vi "Process Mouse Up.vi"(0 "Listbox":refnum<vi>, 1 "Ring":refnum<vi>, 5 "Rows":T1[](array[typedef]), 7 "Items":i32[](array[numeric]), 9 "Coords":T3, 11 "error in (no error)":errorcluster) -> (8 "row":i32, 15 "error out":errorcluster)   [LabVIEW 2015, in "KPropertyTable.xctl"]
uses:
  KPropertyTable.xctl
  <vilib>/Utility/miscctls.llb/LVPoint32TypeDef.ctl
  RowData.ctl
  DataType.ctl
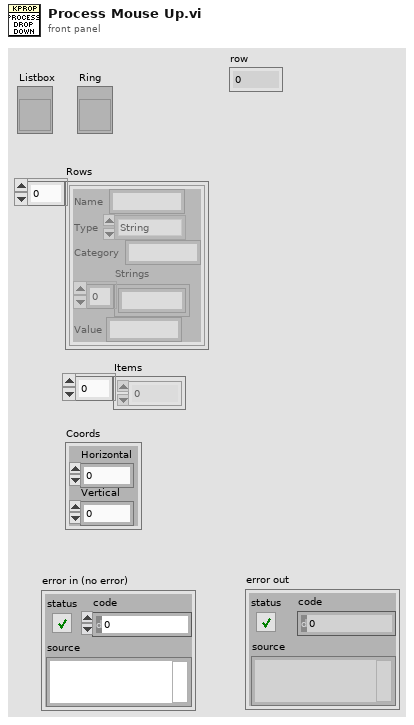
[diagram p1: front panel]
types:
  T1 = typedef "KPropertyTable.xctl/RowData.ctl" = cluster{"Name":string, "Type":T2, "Category":string, "Strings":string[], "Value":string}
  T2 = typedef "KPropertyTable.xctl/DataType.ctl" = enum16{"String", "Enum", "Int", "Double", "Boolean", "Ring", "Formula"}
  T3 = typedef "LVPoint32TypeDef.ctl" = cluster{"Horizontal":i32, "Vertical":i32}
  T4 = typedef "LVRowAndColumnTypeDef.ctl" = cluster{"Row":i32, "Column":i32}
  T5 = typedef "LVPositionTypeDef.ctl" = cluster{"Left":i32, "Top":i32}
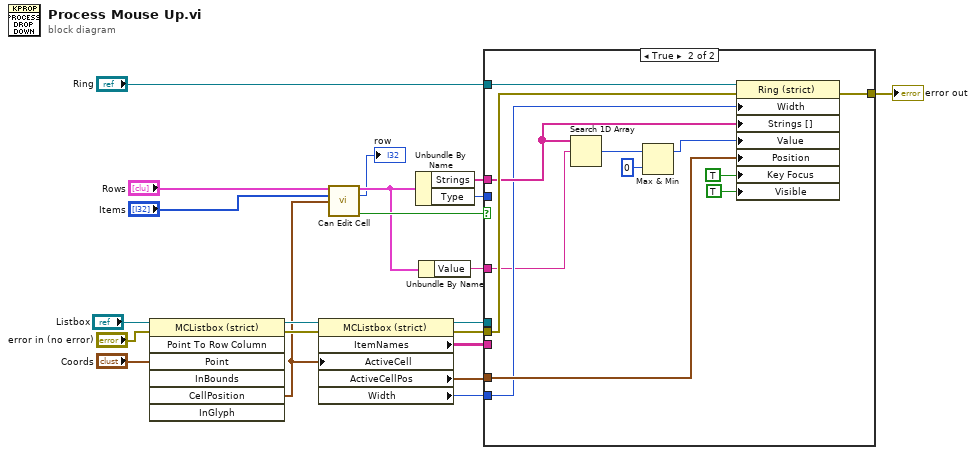
[diagram p0: block diagram]
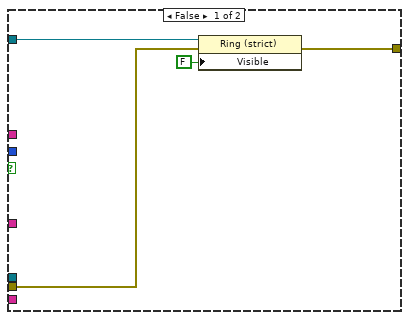
[diagram p2: hidden frame]
diagram:
  n1 = invoke on="Invoke Node" class="MCListbox (strict)" method="Point To Row Column"(reference="Listbox", error in="error in (no error)", "Point"="Coords") -> (reference out=w18:refnum<vi>, error out=w17:errorcluster, "CellPosition"=w7:T4)  [unwired: 4 in, 4 out]
  n2 = property class="MCListbox (strict)"(reference=w18, error in=w17, "ActiveCell"=w7) -> (reference out=w8:refnum<vi>, error out=w12:errorcluster, "ItemNames"=w13:string[][], "ActiveCellPos"=w15:T5, "Width"=w4:u32)
  n3 = call "Can Edit Cell.vi"("Rows"="Rows", "Items"="Items", "Cell"=w7) -> ("item"=w3:T1, "row"=→"row":i32, "enum?"=w5:bool)  [unwired: 9 in, 1 out]
  n4 = Unbundle By Name(w3) -> ("Strings"=w14:string[], "Type"=w10:T2)
  n5 = Unbundle By Name(w3) -> ("Value"=w2:string)
  n6 = case shown="True" w5 {
    tunnel: "Ring" -> [w24 w35]
    tunnel: w15 -> [_ w33]
    tunnel: w14 -> [_ w28]
    tunnel: w13 -> [_ _]
    tunnel: w12 -> [w23 w32]
    tunnel: [w22 w31] -> w11
    tunnel: w10 -> [_ _]
    tunnel: w8 -> [_ _]
    tunnel: w4 -> [_ w27]
    tunnel: w2 -> [_ w26]
    frame False {
      n7 = property on="Property Node" class="Ring (strict)"(reference=w24, error in=w23, "Visible"=FALSE) -> (error out=w22:errorcluster)  [unwired: 1 out]
    }
    frame True {
      n8 = Search 1D Array(1D array=w28, element=w26) -> (index of element=w29:i32)  [unwired: 1 in]
      n9 = Max & Min(x=w29, y=0) -> (max(x,y)=w30:i32)  [unwired: 1 out]
      n10 = property on="Property Node" class="Ring (strict)"(reference=w35, error in=w32, "Width"=w27, "Strings []"=w28, "Value"=w30, "Position"=w33, "Key Focus"=TRUE, "Visible"=TRUE) -> (error out=w31:errorcluster)  [unwired: 1 out]
    }
  }
  "error out" <- w11
